vi "DC bias setting.vi"(2 "VISA resource name":refnum<visa-resource-name>="GPIB12::28::INSTR", 3 "Assign  DC bias according to the chart on the right":dbl=4.0) -> (0 "Send string":string, 1 "Read out result":string)   [LabVIEW 2016]
panel:
  in  "byte count":u32=128
  out "error out":errorcluster {"code" format="%.0x"}
  in  "error in":errorcluster {"code" format="%.0x"}
  # "DC bias enable setting"
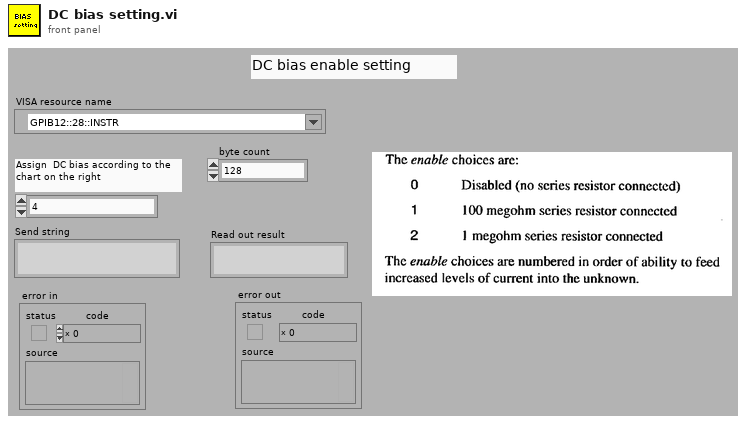
[diagram p1: front panel]
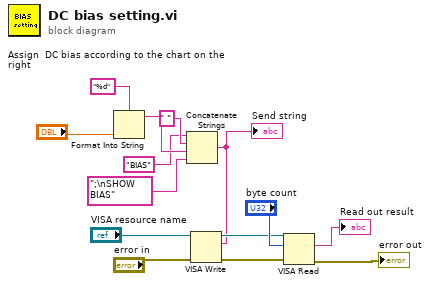
[diagram p0: block diagram]
diagram:
  n1 = Format Into String(format string="%d", "Assign  DC bias according to the chart on the right") -> (resulting string=w10:string)  [unwired: 2 in, 1 out]
  n2 = Concatenate Strings("BIAS" ("string"), " " ("string"), w10, ";\nSHOW BIAS" ("format string")) -> (w3:string)
  "Send string" <- w3
  n3 = VISA Write(VISA resource name="VISA resource name", write buffer=w3, error in (no error)="error in") -> (VISA resource name out=w6:refnum<visa-resource-name>, error out=w5:errorcluster)  [unwired: 1 out]
  n4 = VISA Read(VISA resource name=w6, byte count="byte count", error in (no error)=w5) -> (read buffer=→"Read out result":string, error out=→"error out":errorcluster)  [unwired: 2 out]
